vi "Create Test Configuration.vi"() -> (0 "error out":errorcluster, 1 "Names":string[](array[string]), 2 "Line Array":T1[](array[typedef]), 3 "Module Configuration":refnum<class "Increment configuration.lvclass">, 4 "Channels":refnum<class "TBM channel.lvclass">[](array[class]), 5 "instance identifier":string)   [LabVIEW 2015, in "Increment tests.lvlib"]
doc: "This VI creates a standard test configuration for other unit tests. It currently creates and adds one line with every datatype to the module configuration."
uses:
  Increment tests.lvlib
  module/configuration/Increment configuration.lvclass
  module/configuration/Line.ctl
  <vilib>/NI/Tag Bus Module Framework/channel/TBM channel.lvclass
  <vilib>/NI/Tag Bus/tag/tag descriptor.lvclass/tag descriptor.ctl
  <vilib>/NI/Configuration Framework/serializable configuration/NISE_CEF_serializable configuration.lvclass
  <vilib>/NI/Tag Bus/tag/tag descriptor.lvclass
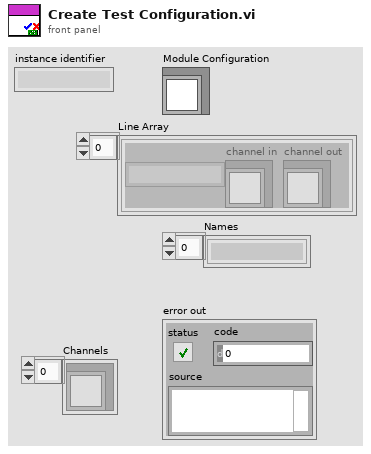
[diagram p1: front panel]
types:
  T1 = typedef "Increment configuration.lvclass/Line.ctl" = cluster{"Name":string, "channel in":refnum<class "TBM channel.lvclass">, "channel out":refnum<class "TBM channel.lvclass">}
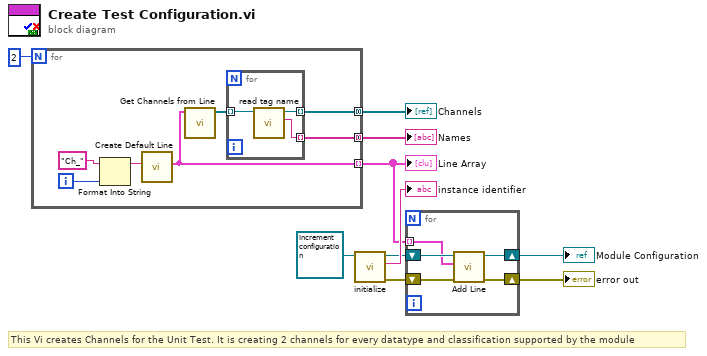
[diagram p0: block diagram]
diagram:
  # "This Vi creates Channels for the Unit Test. It is creating 2 channels for every datatype and classification supported by the module"
  n1 = for {
    N: 2 -> [_]
    tunnel: [w15] -> w6 mode=indexing
    tunnel: [w12] -> w2 mode=concatenating
    tunnel: [w13] -> w7 mode=concatenating
    i -> [w17]
    n2 = Format Into String(initial string="Ch_", w17) -> (resulting string=w11:string)  [unwired: 2 in, 1 out]
    n3 = call "Create Default Line.vi"("Line Name"=w11) -> ("output cluster"=w15:T1)  [unwired: 10 in]
    n4 = call "Get Channels from Line.vi"("Line"=w15) -> ("Channels"=w14:refnum<class "TBM channel.lvclass">[])  [unwired: 10 in]
    n5 = for {
      tunnel: w14 -> [w20] mode=indexing
      tunnel: [w19] -> w13 mode=indexing
      tunnel: [w18] -> w12 mode=indexing
      n6 = call <vilib>:"read tag name.vi"("system tag in"=w20) -> ("name"=w19:string, "system tag out"=w18:refnum<class "TBM channel.lvclass">)  [unwired: 8 in, 1 out]
    }
  }
  "Names" <- w7
  "Line Array" <- w6
  "Channels" <- w2
  n7 = call <vilib>:"initialize.vi"("configuration in"=refnum<class "Increment configuration.lvclass"> refnum ("tag bus configurable plugin module configuration")) -> ("error out"=w8:errorcluster, "identifier"=→"instance identifier":string, "configuration out"=w3:refnum<class "Increment configuration.lvclass">)  [unwired: 8 in]
  n8 = for {
    tunnel: w6 -> [w21] mode=indexing
    shift-right: [w24] -> w5
    shift-left: w3 -> [w25]
    shift-right: [w22] -> w10
    shift-left: w8 -> [w23]
    n9 = call "Add Line.vi"("error in"=w23, "Line"=w21, "Increment configuration in"=w25) -> ("error out"=w22:errorcluster, "Increment configuration out"=w24:refnum<class "Increment configuration.lvclass">)  [unwired: 6 in, 1 out]
  }
  "error out" <- w10
  "Module Configuration" <- w5
